vi "Construct.vi"(8 "Error in (no error)":errorcluster, 10 "Format":string="%Timestamp% %PriorityName% (%Priority%): %Message%") -> (0 "Error out":errorcluster, 3 "LogFormatterSimple out":refnum<class "LogFormatterSimple.lvclass">)   [LabVIEW 2011, in "LogFormatterSimple.lvclass"]
uses:
  LogFormatterSimple.lvclass
  LogFormatterSimple.lvclass/LogFormatterSimple.ctl
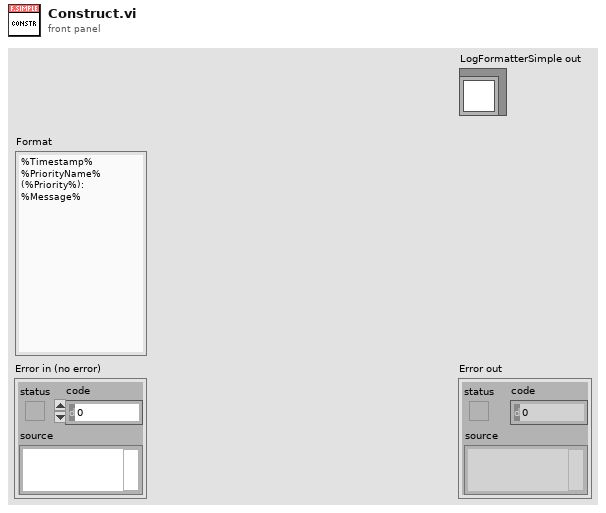
[diagram p1: front panel]
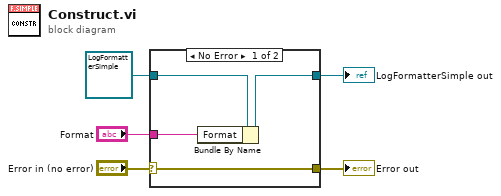
[diagram p0: block diagram]
diagram:
  n1 = case shown="No Error" "Error in (no error)" {
    selector: "Error in (no error)" -> [w9 w11]
    tunnel: [w9 w11] -> w4
    tunnel: [w7 w10] -> w3
    tunnel: refnum<class "LogFormatterSimple.lvclass"> refnum ("LogFormatterSimple in") -> [w8 w10]
    tunnel: "Format" -> [w6 _]
    frame No Error {
      n2 = Bundle By Name(cluster=w8, "Format"=w6) -> (w7:refnum<class "LogFormatterSimple.lvclass">)
    }
    frame Error {
    }
  }
  "Error out" <- w4
  "LogFormatterSimple out" <- w3
